vi "do_povorota.vi"() -> ()   [LabVIEW 2017]
uses:
  <vilib>/userdefined/High Color/IMAQdx.ctl
  <vilib>/myRIO/Instrument Drivers/Onboard IO/PWM/typedefs/PWM Reference.ctl
  <vilib>/myRIO/Common/Instrument Driver Framework/Utilities/typedefs/myRIO Generic Hardware Reference.ctl
  <vilib>/myRIO/Common/Instrument Driver Framework/Utilities/typedefs/Hardware Version Enum.ctl
  <vilib>/myRIO/Common/Instrument Driver Framework/Utilities/typedefs/myRIO v1.0 Reference.ctl
  <vilib>/myRIO/Common/Instrument Driver Framework/Utilities/typedefs/Generic FPGA Reference.ctl
  <vilib>/myRIO/Common/Instrument Driver Framework/myRIO v1.0/PWM/typedefs/PWM Channels Enum.ctl
  <vilib>/myRIO/Instrument Drivers/Onboard IO/PWM/typedefs/PWM Configuration.ctl
  <vilib>/userdefined/High Color/nirio_resource_hc.ctl
  <vilib>/myRIO/Common/Instrument Driver Framework/Utilities/vis/Is FPGA Ref Available.vi
  <vilib>/myRIO/Common/Instrument Driver Framework/myRIO v1.0/PWM/vis/myRIO v1.1 Open PWM.vi
  <vilib>/myRIO/Instrument Drivers/Onboard IO/PWM/vis/Set Duty Cycle and Frequency.vi
  <vilib>/myRIO/Common/Instrument Driver Framework/Utilities/vis/Validate Channels.vi
  <vilib>/myRIO/Common/Instrument Driver Framework/myRIO v1.0/PWM/vis/myRIO v1.0 Reserve PWM.vi
  <vilib>/myRIO/Common/Instrument Driver Framework/myRIO v1.0/PWM/vis/myRIO v1.0 Build MUX Configuration PWM.vi
  <vilib>/myRIO/Common/Instrument Driver Framework/myRIO v1.0/Resource Manager/vis/myRIO v1.0 Reserve Channel List.vi
  <vilib>/myRIO/Common/Instrument Driver Framework/myRIO v1.0/Resource Manager/vis/myRIO v1.0 Create Configuration List.vi
  <vilib>/myRIO/Common/Instrument Driver Framework/myRIO v1.0/Resource Manager/vis/myRIO v1.0 Reserve Channel.vi
  <vilib>/myRIO/Common/Instrument Driver Framework/myRIO v1.0/Resource Manager/vis/myRIO v1.0 Unreserve Channel.vi
  <vilib>/myRIO/Common/Instrument Driver Framework/myRIO v1.0/Resource Manager/vis/myRIO v1.0 Build Mutex Name.vi
  <vilib>/Utility/VariantDataType/GetNumericInfo.vi
  <vilib>/Utility/error.llb/Error Cluster From Error Code.vi
  <vilib>/myRIO/Common/Instrument Driver Framework/myRIO v1.0/myRIO v1.1 Open.vi
  <vilib>/myRIO/Common/Instrument Driver Framework/Utilities/vis/IO Manager.vi
  <vilib>/myRIO/Common/Instrument Driver Framework/Utilities/vis/Configuration Manager.vi
  <vilib>/myRIO/Common/Instrument Driver Framework/myRIO v1.0/Resource Manager/vis/myRIO v1.0 Configure IO.vi
  <vilib>/myRIO/Common/Instrument Driver Framework/myRIO v1.0/myRIO v1.0 Close.vi
  <vilib>/myRIO/Common/Instrument Driver Framework/myRIO v1.0/PWM/vis/myRIO v1.0 Write PWM.vi
  <vilib>/myRIO/Express VI/Onboard IO/PWM/PWM Express VI.xnode
  <vilib>/myRIO/Instrument Drivers/Onboard IO/PWM/vis/myRIO PWM Open.xnode
  <vilib>/vision/driver/NI_Vision_Acquisition_Software.lvlib
  <vilib>/myRIO/Instrument Drivers/Onboard IO/PWM/PWM.lvlib
panel:
  out "stop":i32
  out "peh":i32
  in  "stop":bool
  out "X":sgl
  # "s"
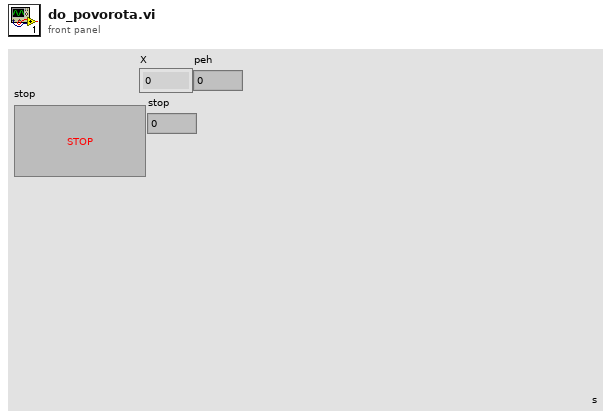
[diagram p1: front panel]
types:
  T1 = typedef "IMAQdx.ctl" = refnum<k21>
  T2 = typedef "IMAQ Image.ctl" = refnum<image>
  T3 = typedef "PWM.lvlib/PWM Reference.ctl" = cluster{"myRIO Reference":T4, "PWM Channels Enum":T8, "PWM Configuration":T9}
  T4 = typedef "myRIO Generic Hardware Reference.ctl" = cluster{"myRIO Model":T5, "myRIO Hardware Reference":T6}
  T5 = typedef "Hardware Version Enum.ctl" = enum16{"Unknown", "myRIO-1900", "myRIO-1950", "roboRIO", "NI ELVIS RIO CM"}
  T6 = typedef "myRIO v1.0 Reference.ctl" = cluster{"Generic FPGA Reference":T7, "Allow multiple opens":bool}
  T7 = typedef "Generic FPGA Reference.ctl" = refnum<k20>
  T8 = typedef "PWM Channels Enum.ctl" = enum16{"Not Connected", "C/PWM0", "C/PWM1", "A/PWM0", "A/PWM1", "A/PWM2", "B/PWM0", "B/PWM1", "B/PWM2", "PWM/PWM0", "PWM/PWM1", "PWM/PWM2", "PWM/PWM3", "PWM/PWM4", "PWM/PWM5", "PWM/PWM6", "PWM/PWM7", "PWM/PWM8", "PWM/PWM9"}
  T9 = typedef "PWM.lvlib/PWM Configuration.ctl" = cluster{"Frequency":dbl, "Duty Cycle":dbl}
  T10 = typedef "nirio_resource_hc.ctl" = tag
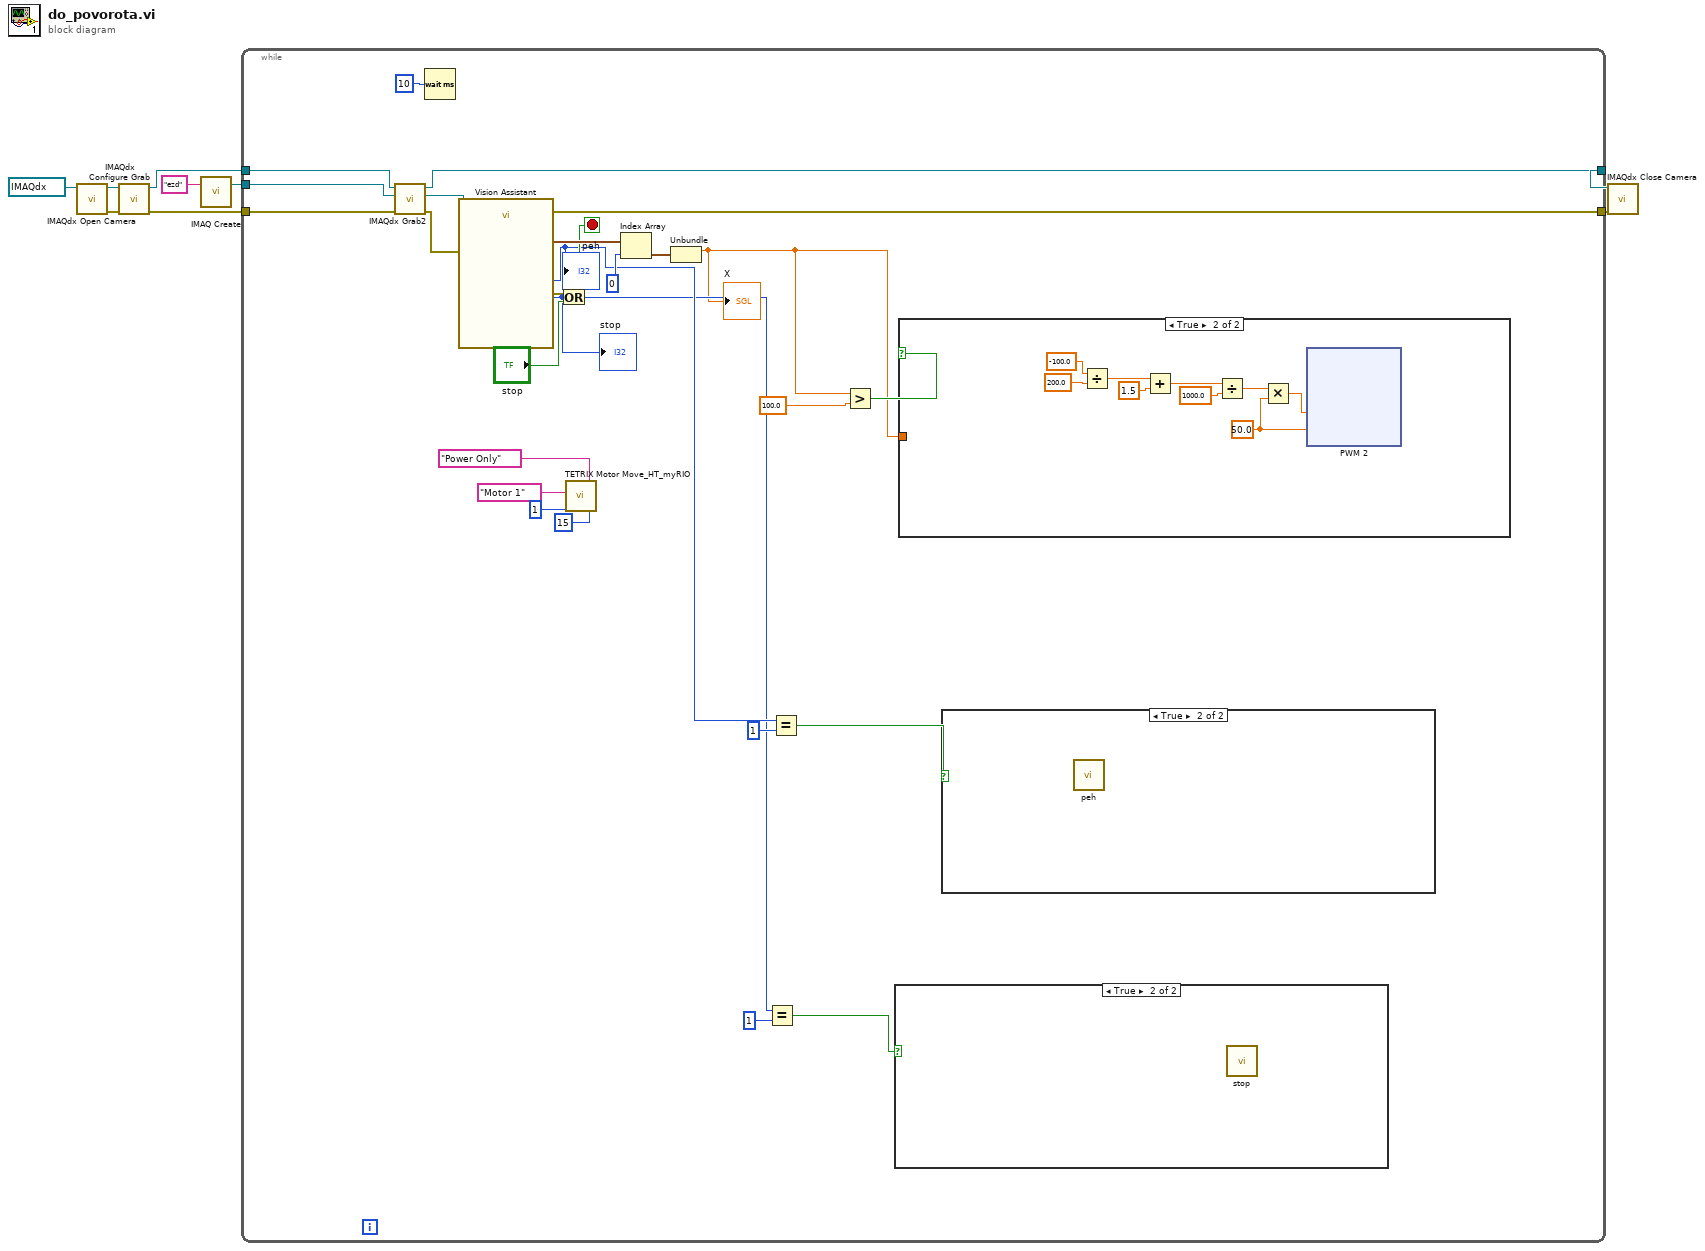
[diagram p0: block diagram]
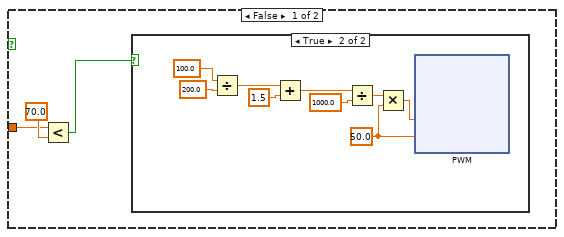
[diagram p4: hidden frame]
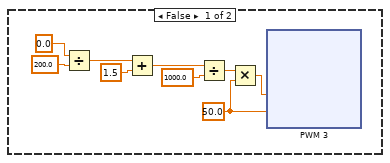
[diagram p5: hidden frame]
diagram:
  n1 = call <vilib>:"IMAQdx Open Camera.vi"("Session In"=T1 "cam0") -> ("error out"=w6:errorcluster, "Session Out"=w7:T1)  [unwired: 9 in]
  n2 = call <vilib>:"IMAQdx Configure Grab.vi"("error in"=w6, "Session In"=w7) -> ("error out"=w5:errorcluster, "Session Out"=w8:T1)  [unwired: 8 in]
  n3 = call "IMAQ Create"("Image Name"="ezd") -> ("New Image"=w9:T2)  [unwired: 4 in, 1 out]
  n4 = while {
    tunnel: w5 -> [w30]
    tunnel: w9 -> [w29]
    tunnel: w8 -> [w28]
    tunnel: [w27] -> w3
    tunnel: [w23] -> w4
    stop <- w22 stop-if-true
    n5 = call <vilib>:"IMAQdx Grab2.vi"("error in"=w30, "Image In"=w29, "Session In"=w28) -> ("error out"=w32:errorcluster, "Image Out"=w31:T2, "Session Out"=w27:T1)  [unwired: 5 in, 1 out]
    n6 = Wait (ms)(milliseconds to wait=u32 10) -> ()  [unwired: 1 out]
    n7 = call "Vision Assistant"("Image In"=w31, "error in"=w32) -> ("Edges Coordinates (Edge Detector 1)"=w35:cluster{"X":sgl, "Y":sgl}[], "Number of Matches (Color Location 2)"=w20:i32, "Number of Matches (Color Location 1)"=w17:i32, "error out"=w23:errorcluster)  [unwired: 20 in, 2 out]
    "peh" <- w20
    "stop" <- w17
    n8 = Or(x=w23, y="stop") -> (x .or. y?=w22:bool)
    n9 = call <vilib>:"TETRIX Motor Move_HT_myRIO.vi"("Power (-100 to 100)\n0 = Stop/Brake\n-128 = Stop/Coast"=i8 15 ("Power (-100 to 100)\n0 = Stop/Brake\n-128 = Stop/Coast"), "Control Mode"="Power Only", "Controller Daisy Chain Position: 1 - 4"=u8 1, "Select Channel"="Motor 1") -> ()  [unwired: 3 in, 1 out]
    n10 = Index Array(array=w35, index=0) -> (element=w34:cluster{"X":sgl, "Y":sgl})
    n11 = Unbundle(w34) -> ("X"=w15:sgl)  [unwired: 1 out]
    "X" <- w15
    n12 = Equal?(x=w17, y=1) -> (x = y?=w14:bool)
    n13 = Equal?(x=w20, y=1) -> (x = y?=w21:bool)
    n14 = Greater?(x=w15, y=sgl 100.0) -> (0:w16:bool)
    n15 = case shown="True" w14 {
      frame False {
      }
      frame True {
        n16 = call "stop.vi"() -> ()  [unwired: 12 in]
      }
    }
    n17 = case shown="True" w16 {
      tunnel: w15 -> [w37 _]
      frame False {
        n18 = Less?(x=w37, y=sgl 70.0) -> (x < y?=w36:bool)
        n19 = case shown="True" w36 {
          frame False {
            w43 = 50.0 ("Frequency [Hz]")
            n20 = Divide(x=0.0, y=200.0) -> (x/y=w46:dbl)
            n21 = Add(x=w46, y=1.5) -> (x+y=w45:dbl)
            n22 = Divide(x=w45, y=1000.0) -> (x/y=w44:dbl)
            n23 = Multiply(x=w44, y=w43) -> (x*y=w47:dbl)
            n24 = xnode "PWM 3"("Duty Cycle"=w47, "Frequency [Hz]"=w43) -> ()  [unwired: 1 in, 1 out]
          }
          frame True {
            w87 = 50.0 ("Frequency [Hz]")
            n25 = Divide(x=100.0, y=200.0) -> (x/y=w90:dbl)
            n26 = Add(x=w90, y=1.5) -> (x+y=w89:dbl)
            n27 = Divide(x=w89, y=1000.0) -> (x/y=w88:dbl)
            n28 = Multiply(x=w88, y=w87) -> (x*y=w91:dbl)
            n29 = xnode "PWM"("Duty Cycle"=w91, "Frequency [Hz]"=w87) -> ()  [unwired: 1 in, 1 out]
          }
        }
      }
      frame True {
        w131 = 50.0 ("Frequency [Hz]")
        n30 = Divide(x=-100.0, y=200.0) -> (x/y=w134:dbl)
        n31 = Add(x=w134, y=1.5) -> (x+y=w133:dbl)
        n32 = Divide(x=w133, y=1000.0) -> (x/y=w132:dbl)
        n33 = Multiply(x=w132, y=w131) -> (x*y=w135:dbl)
        n34 = xnode "PWM 2"("Duty Cycle"=w135, "Frequency [Hz]"=w131) -> ()  [unwired: 1 in, 1 out]
      }
    }
    n35 = case shown="True" w21 {
      frame False {
      }
      frame True {
        n36 = call "peh.vi"() -> ()  [unwired: 12 in]
      }
    }
  }
  n37 = call <vilib>:"IMAQdx Close Camera.vi"("error in"=w4, "Session In"=w3) -> ()  [unwired: 9 in, 1 out]
